vi "Host - Seggregate DO names.vi"(9 "Co-Pilot Control Names":string[][](array[string]), 10 "Pilot Control Names":string[](array[string]), 11 "GUI Data":string[](array[string])) -> (1 "Co-Pilot DO":cluster{"Data":i32[]}[](array[cluster]), 2 "Pilot DO":cluster{"Data":i32[]}[](array[cluster]))   [LabVIEW 2021]
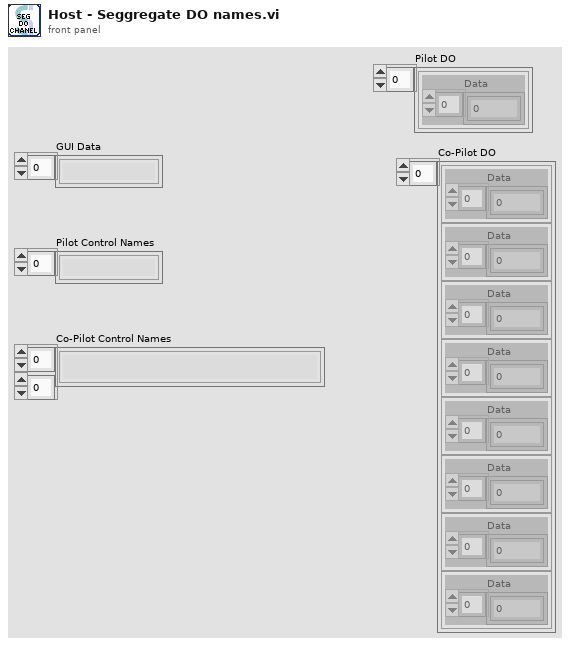
[diagram p1: front panel]
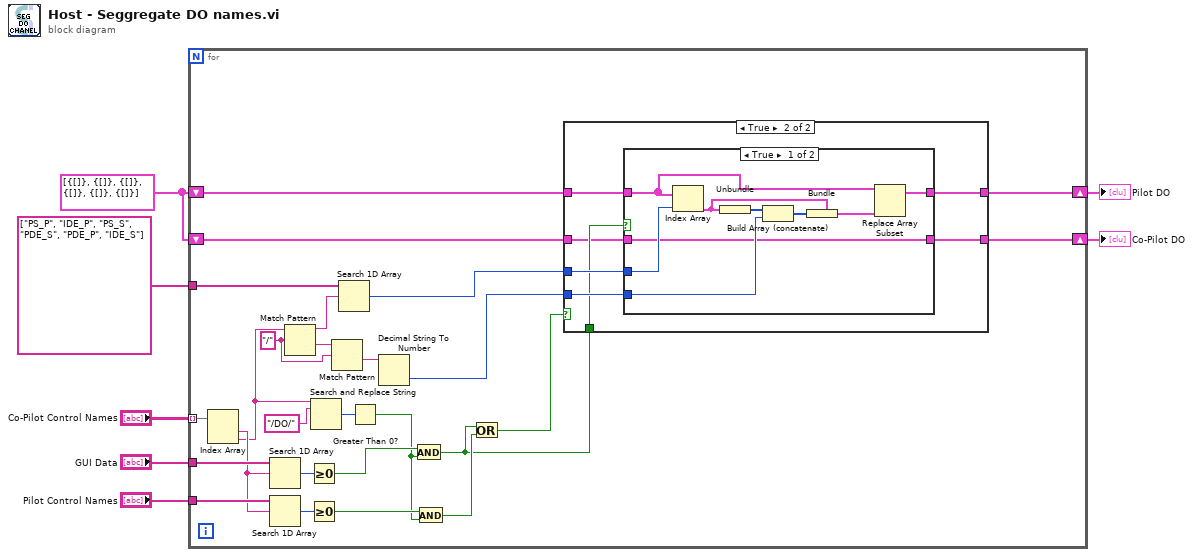
[diagram p0: block diagram]
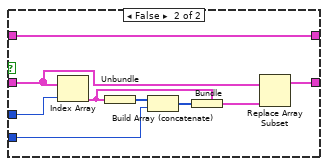
[diagram p3: hidden frame]
diagram:
  w1 = cluster{"Data":i32[]}[] [{"Data"=[]}, {"Data"=[]}, {"Data"=[]}, {"Data"=[]}, {"Data"=[]}, {"Data"=[]}] ("initialized array")
  n1 = for {
    tunnel: "Co-Pilot Control Names" -> [w33] mode=indexing
    tunnel: "Pilot Control Names" -> [w31]
    tunnel: "GUI Data" -> [w32]
    tunnel: string[] ["PS_P", "IDE_P", "PS_S", "PDE_S", "PDE_P", "IDE_S"] ("Addresses") -> [w21]
    shift-right: [w8] -> w3
    shift-left: w1 -> [w14]
    shift-right: [w9] -> w2
    shift-left: w1 -> [w10]
    w18 = "/" ("regular expression")
    n2 = Index Array(array=w33) -> (element #1=w30:string, element #2=w22:string)  [unwired: 2 in]
    n3 = Search 1D Array(1D array=w32, element=w30) -> (index of element=w29:i32)  [unwired: 1 in]
    n4 = Search 1D Array(1D array=w31, element=w30) -> (index of element=w28:i32)  [unwired: 1 in]
    n5 = Match Pattern(string=w22, regular expression=w18) -> (before substring=w20:string, after substring=w19:string)  [unwired: 1 in, 2 out]
    n6 = Greater Or Equal To 0?(x=w29) -> (x >= 0?=w27:bool)
    n7 = Greater Or Equal To 0?(x=w28) -> (x >= 0?=w26:bool)
    n8 = Search and Replace String(input string=w22, search string="/DO/") -> (number of replacements=w24:i32)  [unwired: 6 in, 3 out]
    n9 = Match Pattern(string=w19, regular expression=w18) -> (after substring=w17:string)  [unwired: 1 in, 3 out]
    n10 = Search 1D Array(1D array=w21, element=w20) -> (index of element=w16:i32)  [unwired: 1 in]
    n11 = Greater Than 0?(x=w24) -> (x > 0?=w23:bool)
    n12 = Decimal String To Number(string=w17) -> (number=w15:i32)  [unwired: 2 in, 1 out]
    n13 = And(x=w27, y=w23) -> (x .and. y?=w11:bool)
    n14 = And(x=w26, y=w23) -> (x .and. y?=w13:bool)
    n15 = Or(x=w11, y=w13) -> (x .or. y?=w12:bool)
    n16 = case shown="True" w12 {
      tunnel: w16 -> [_ w42]
      tunnel: w15 -> [_ w41]
      tunnel: w14 -> [w35 w40]
      tunnel: w11 -> [_ w38]
      tunnel: w10 -> [w34 w37]
      tunnel: [w35 w39] -> w8
      tunnel: [w34 w36] -> w9
      frame False {
      }
      frame True {
        n17 = case shown="True" w38 {
          tunnel: w42 -> [w51 w60]
          tunnel: w41 -> [w49 w58]
          tunnel: w40 -> [w45 w52]
          tunnel: [w44 w52] -> w39
          tunnel: w37 -> [w43 w53]
          tunnel: [w43 w54] -> w36
          frame True {
            n18 = Index Array(array=w45, index=w51) -> (element=w47:cluster{"Data":i32[]})
            n19 = Unbundle(w47) -> ("Data"=w50:i32[])
            n20 = Build Array (concatenate)(w50, w49) -> (w48:i32[])
            n21 = Bundle(cluster=w47, "Data"=w48) -> (w46:cluster{"Data":i32[]})
            n22 = Replace Array Subset(array=w45, new element=w46) -> (w44:cluster{"Data":i32[]}[])  [unwired: 1 in]
          }
          frame False {
            n23 = Index Array(array=w53, index=w60) -> (element=w56:cluster{"Data":i32[]})
            n24 = Unbundle(w56) -> ("Data"=w59:i32[])
            n25 = Build Array (concatenate)(w59, w58) -> (w57:i32[])
            n26 = Bundle(cluster=w56, "Data"=w57) -> (w55:cluster{"Data":i32[]})
            n27 = Replace Array Subset(array=w53, new element=w55) -> (w54:cluster{"Data":i32[]}[])  [unwired: 1 in]
          }
        }
      }
    }
  }
  "Pilot DO" <- w3
  "Co-Pilot DO" <- w2
